vi "Read_Data_file_old.vi"(0 "Results file":path, 1 "Read Channel Names only":bool, 3 "Add Extra Channels?":bool, 5 "Template File":path, 8 "Read Results file only?":bool) -> (10 "Row numbers":i32[](array[numeric]), 11 "Template File Out":path, 12 "Filetype":string, 13 "EOF?":bool, 14 "Results file Out":path, 15 "String Before":string, 16 "Ch names Out":string[](array[string]), 17 "Channel Values Out":string[][](array[string]), 18 "String After":string, 19 "mark after read (chars.)":i32)   [LabVIEW 2010]
uses:
  Results_plotter_Global.vi
  Globals/Meas_global.vi
panel:
  out "Case":string
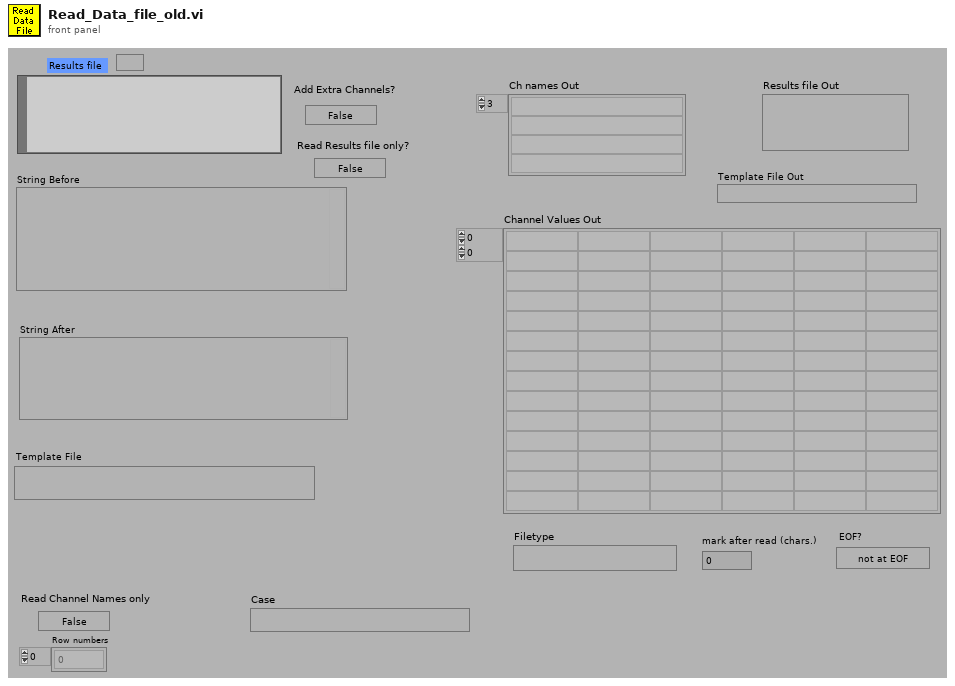
[diagram p1: front panel]
types:
  T1 = enum32{"existing file", "new file", "new or existing file", "existing dir", "new dir", "new or existing dir", "existing file (use LLBs)", "new file (use LLBs)", "new or existing file (use LLBs)", "new or existing file or directory (use LLBs)"}
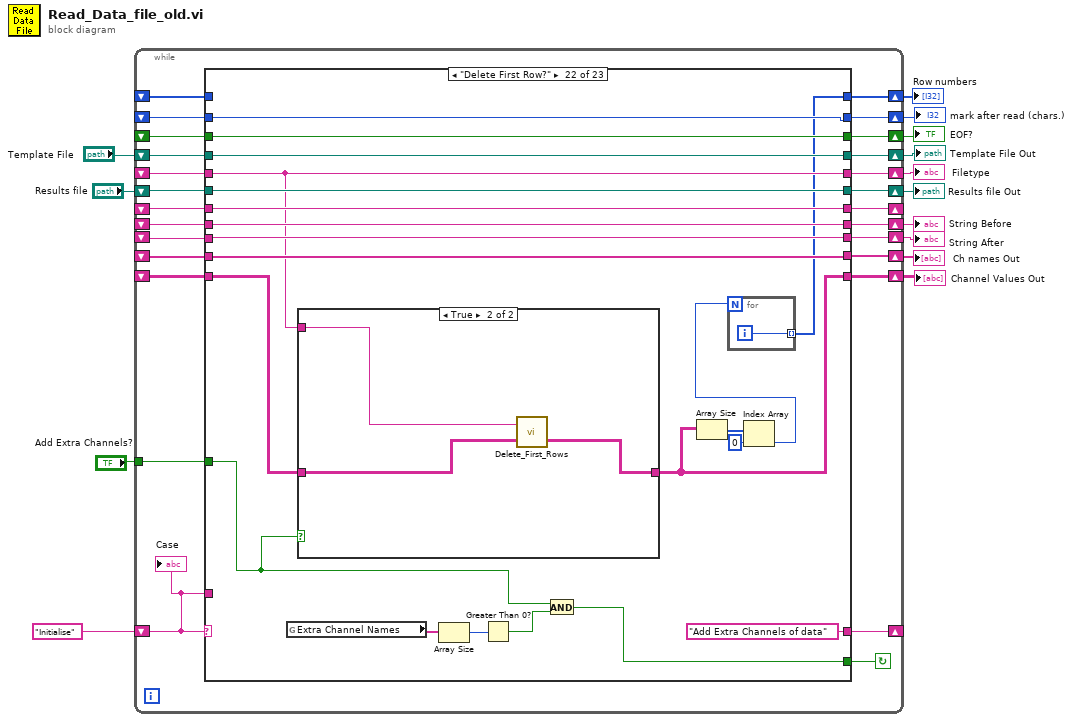
[diagram p0: block diagram]
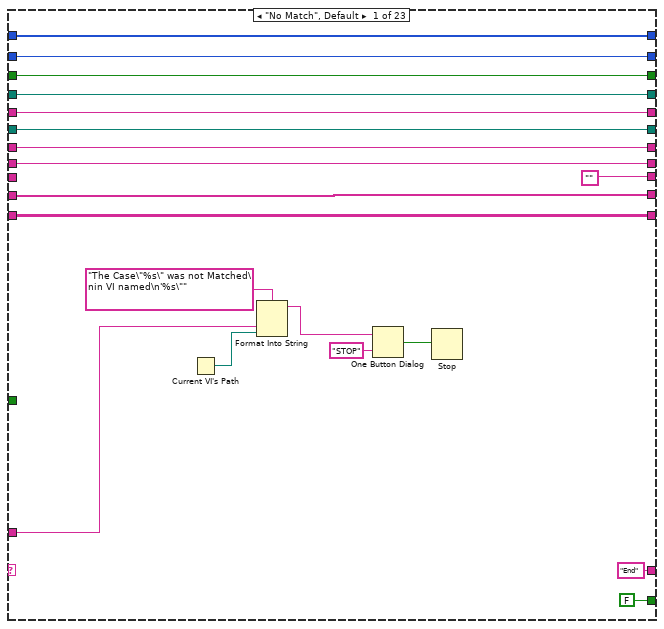
[diagram p2: hidden frame]
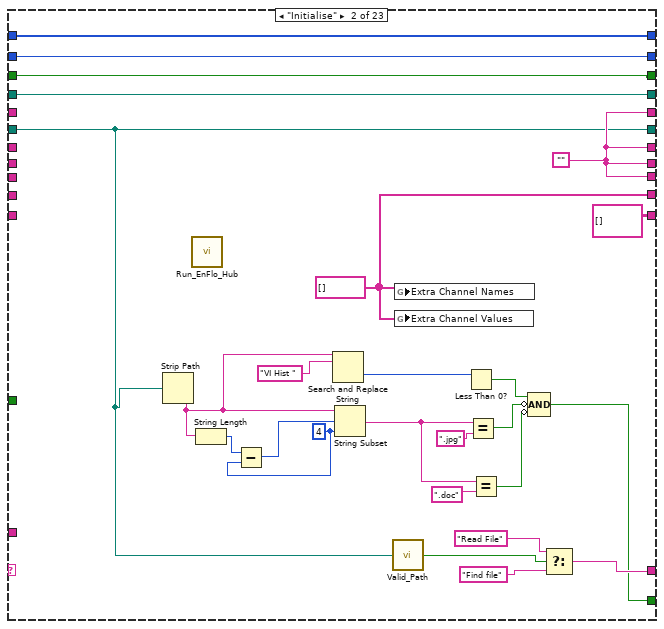
[diagram p3: hidden frame]
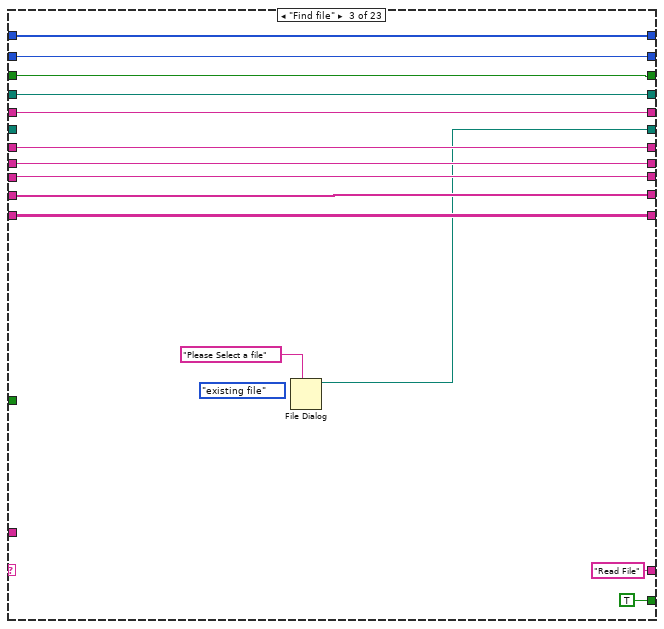
[diagram p4: hidden frame]
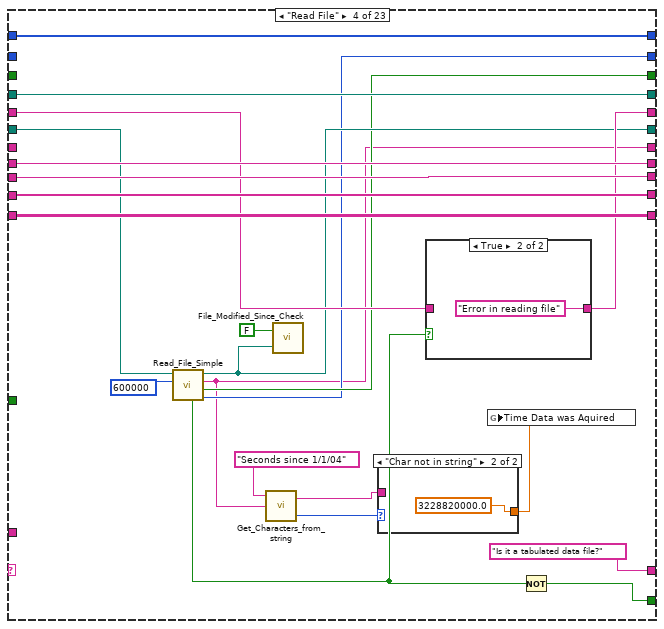
[diagram p5: hidden frame]
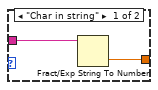
[diagram p6: hidden frame]
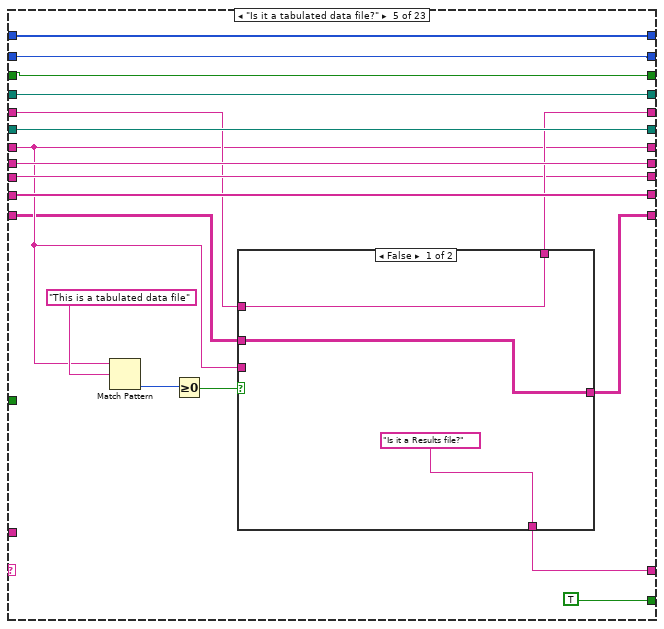
[diagram p8: hidden frame]
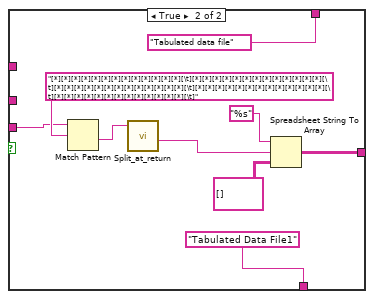
[diagram p9: hidden frame]
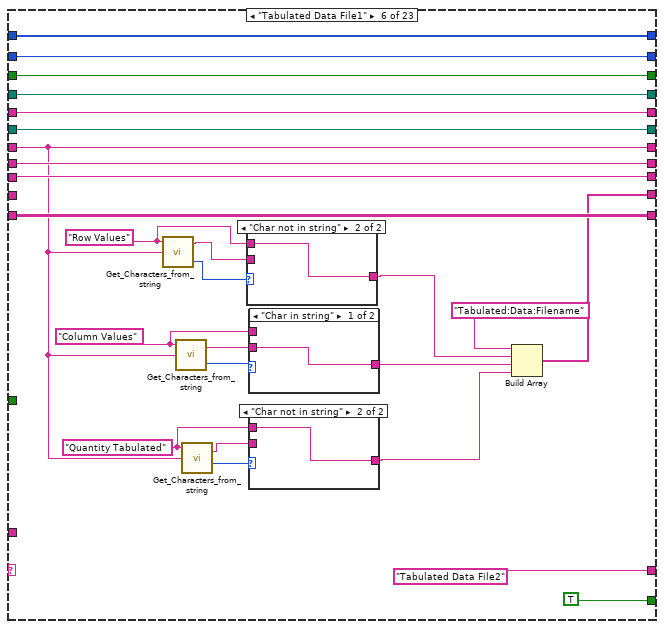
[diagram p10: hidden frame]
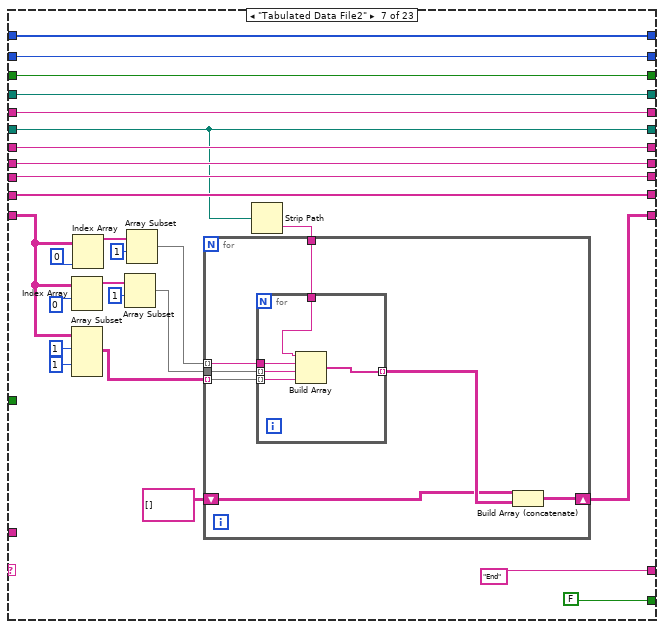
[diagram p14: hidden frame]
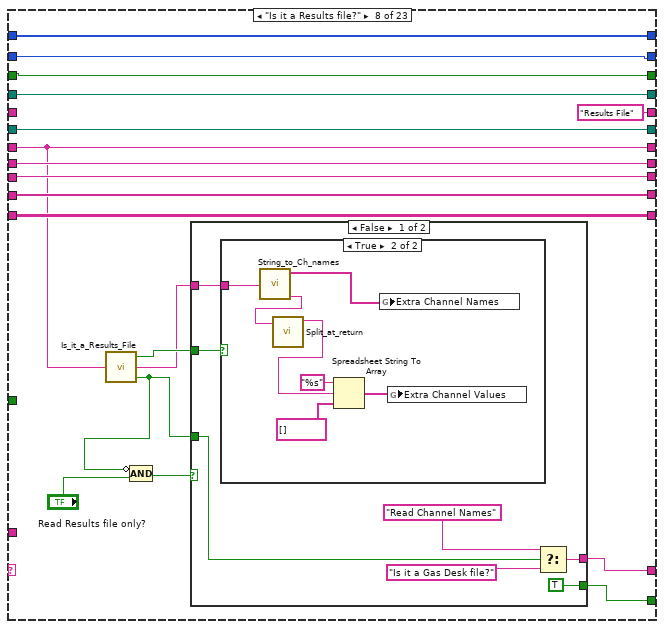
[diagram p15: hidden frame]
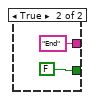
[diagram p17: hidden frame]
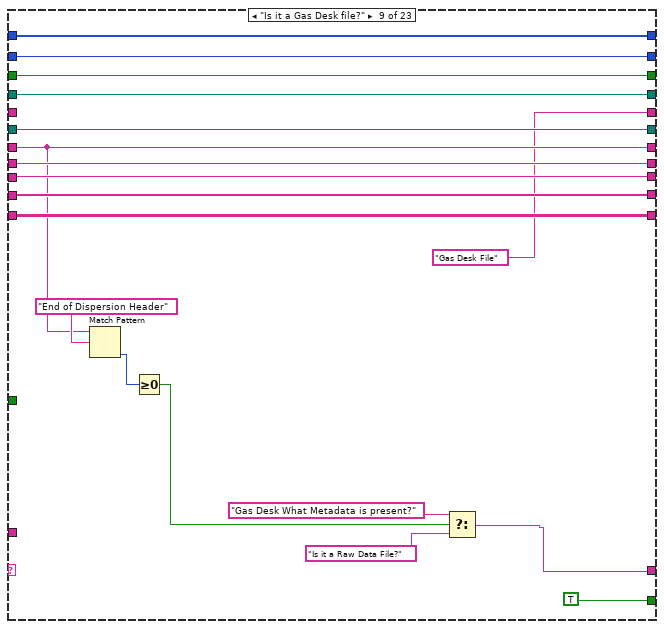
[diagram p18: hidden frame]
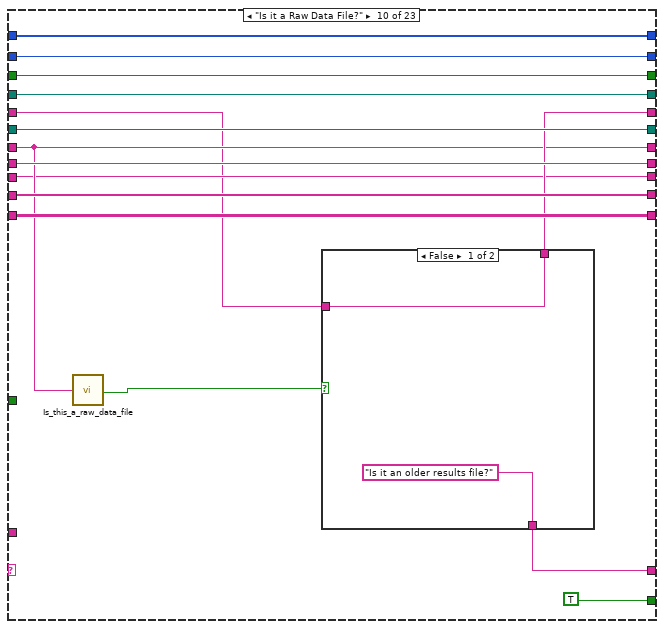
[diagram p19: hidden frame]
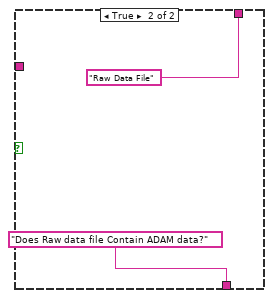
[diagram p20: hidden frame]
diagram:
  n1 = while {
    tunnel: "Add Extra Channels?" -> [w23]
    shift-left: _ -> [w27]
    shift-right: [w26] -> w13
    shift-left: "Results file" -> [w29]
    shift-right: [w28] -> w11
    shift-left: _ -> [w31]
    shift-right: [w30] -> w6
    shift-left: _ -> [w24]
    shift-right: [w32] -> w8
    shift-left: _ -> [w33]
    shift-right: [w34] -> _
    shift-left: "Initialise" -> [w37]
    shift-right: [w35] -> _
    shift-left: _ -> [w25]
    shift-right: [w39] -> w9
    shift-left: _ -> [w36]
    shift-right: [w40] -> w10
    shift-right: [w22] -> w5
    shift-left: "Template File" -> [w21]
    shift-right: [w19] -> w3
    shift-left: _ -> [w20]
    shift-right: [w18] -> w2
    shift-left: _ -> [w17]
    shift-right: [w15] -> w1
    shift-left: _ -> [w16]
    stop <- w38 continue-if-true
    n2 = case shown="\"Delete First Row?\"" w37 {
      tunnel: [w52 w83 w97 w119 w143 w163 w214 w244 w278 w293 w314 w339 w366 w387 w426 w454 w467 w529 w552 w588 w614 w646 w665] -> w40
      tunnel: [w51 string[][] [] ("Channel Values") w96 w118 w131 w181 w203 w243 w277 w292 w313 w338 w365 w386 w425 w453 w475 w535 w577 w587 w609 w635 w661] -> w39
      tunnel: [FALSE ("Results File?") w72 TRUE ("Results File?") w115 TRUE ("Results File?") TRUE ("Results File?") FALSE ("Results File?") w235 TRUE ("Results File?") TRUE ("Results File?") TRUE ("Results File?") w324 w358 TRUE ("Results File?") TRUE ("Results File?") TRUE ("Results File?") w461 TRUE ("Results File?") TRUE ("Results File?") FALSE ("Results File?") TRUE ("Results File?") w640 FALSE ("Results File?")] -> w38
      tunnel: w37 -> [w54 _ _ _ _ _ _ _ _ _ _ _ _ _ _ _ _ _ _ _ _ _ _]
      tunnel: w36 -> [w52 _ w97 w119 w143 _ w214 w244 w278 w293 w314 w339 w366 w387 w426 w454 _ w529 w553 w592 w614 w646 w668]
      tunnel: ["End" w84 "Read File" "Is it a tabulated data file?" w138 "Tabulated Data File2" ("f") "End" ("f") w242 w265 w287 w308 "Read Channel Names" ("f") "Read Channel Names" ("f") w372 "Read Channel Names" ("f") "Read Channel Names" ("f") w465 "Does template file exist?" ("f") w572 "End" ("f") "Delete First Row?" ("f") "Add Extra Channels of data" ("f") "End" ("f")] -> w35
      tunnel: [w49 w81 w94 w101 w132 w174 w210 w237 w271 w285 w303 w333 w354 w374 w404 w437 w468 w530 w576 w593 w607 w648 w670] -> w34
      tunnel: w33 -> [w49 _ w94 _ w132 w174 w210 w237 w271 w285 w303 w333 w361 w373 w404 w437 w470 w530 w576 w593 w607 w648 w670]
      tunnel: [w48 w81 w93 w117 w141 w179 w213 w238 w274 w290 w311 w336 w363 w383 w422 w451 w469 w527 w575 w596 w613 w651 w674] -> w32
      tunnel: w31 -> [_ _ w92 w116 w137 w177 w211 w240 w275 w284 w307 w335 _ w384 w423 w452 w474 w534 w574 w595 w612 w650 w673]
      tunnel: ["" w81 w92 w116 w137 w177 w211 w240 w275 w284 w307 w335 w351 w384 w423 w452 w474 w534 w574 w595 w612 w650 w673] -> w30
      tunnel: w29 -> [w47 w65 _ w112 w142 w180 w193 w241 w276 w291 w312 w337 w364 w385 w424 w431 w473 w533 w570 w591 w606 w647 w669]
      tunnel: [w47 w65 w91 w108 w142 w180 w193 w241 w276 w291 w312 w337 w364 w385 w424 w431 w473 w533 w570 w591 w606 w647 w669] -> w28
      tunnel: w27 -> [w45 _ w89 w113 w136 w176 w209 _ _ w283 w306 _ w357 w371 w420 w449 w472 w532 w573 w590 w603 w645 w672]
      tunnel: [w45 w81 w89 w114 w139 w176 w209 "Results File" "Gas Desk File" w288 w309 w323 w357 w371 w420 w449 w472 w532 w573 w590 w603 w645 w672] -> w26
      tunnel: w25 -> [w51 _ w96 w118 w130 w181 w202 w243 w277 w292 w313 w338 w365 w386 w425 w453 w475 w535 w577 _ _ w644 w663]
      tunnel: w24 -> [w48 _ w93 w117 w141 w179 w213 w238 w274 w290 w311 w336 w363 w383 w422 w451 _ w527 w575 w596 w613 w651 w674]
      tunnel: w23 -> [_ _ _ _ _ _ _ _ _ _ _ w325 _ _ _ _ _ _ _ _ _ w639 _]
      tunnel: [w44 w71 w88 w107 w129 w159 w191 w231 w264 w282 w301 w322 w348 w370 w402 w430 w463 w525 w555 w586 w602 w638 w660] -> w22
      tunnel: w21 -> [w44 w71 w88 w107 w129 w159 w191 w231 w264 w282 w301 w322 w348 w370 w402 w430 w463 w525 w555 w585 w602 w638 w660]
      tunnel: w20 -> [w42 w69 w86 _ w127 w157 w189 w229 w262 w280 w299 w320 w346 w368 w400 w428 w462 w524 w564 w584 w601 w636 w658]
      tunnel: [w42 w69 w86 w106 w127 w157 w189 w229 w262 w280 w299 w320 w346 w368 w400 w428 w462 w524 w564 w584 w600 w636 w658] -> w19
      tunnel: [w43 w70 w87 w105 w128 w158 w190 w230 w263 w281 w300 w321 w347 w369 w401 w429 w458 w523 w563 w583 w599 w637 w659] -> w18
      tunnel: w17 -> [w43 w70 w87 _ w128 w158 w190 w230 w263 w281 w300 w321 w347 w369 w401 w429 w459 w523 w563 w583 w599 w637 w659]
      tunnel: [w41 w68 w85 w104 w126 w156 w188 w228 w261 w279 w298 w319 w345 w367 w399 w427 w455 w522 w562 w582 w598 w631 w657] -> w15
      tunnel: w16 -> [w41 w68 w85 w104 w126 w156 w188 w228 w261 w279 w298 w319 w345 w367 w399 w427 w455 w522 w562 _ w598 _ w657]
      frame "No Match", Default {
        n3 = Current VI's Path() -> (path=w55:path)
        n4 = Format Into String(format string="The Case\"%s\" was not Matched\nin VI named\n'%s\"" ("Format String"), w54, w55) -> (resulting string=w58:string)  [unwired: 2 in, 1 out]
        n5 = One Button Dialog(message=w58, button name ("OK")="STOP") -> (true=w56:bool)
        n6 = Stop(stop? (T)=w56) -> ()
      }
      frame "Initialise" {
        w79 = 4 ("length (rest)")
        w81 = ""
        w83 = string[] [] ("Extra Channel Names")
        n7 = Strip Path(path=w65) -> (name=w77:string)  [unwired: 1 out]
        n8 = call "Run_EnFlo_Hub.vi"() -> ()  [unwired: 8 in]
        n9 = String Length(string=w77) -> (length=w80:i32)
        n10 = Subtract(x=w80, y=w79) -> (x-y=w78:i32)
        n11 = Search and Replace String(input string=w77, search string="VI Hist ") -> (offset past replacement=w75:i32)  [unwired: 6 in, 3 out]
        n12 = String Subset(string=w77, offset (0)=w78, length (rest)=w79) -> (substring=w62:string)
        n13 = call "Valid_Path.vi"("Filename"=w65) -> ("Valid Path?"=w64:bool)
        n14 = global write "Results_plotter_Global.vi" "Extra Channel Names"(w83) -> ()
        n15 = global write "Results_plotter_Global.vi" "Extra Channel Values"(w83) -> ()
        n16 = Less Than 0?(x=w75) -> (x < 0?=w73:bool)
        n17 = Equal?(x=w62, y=".jpg") -> (x = y?=w74:bool)
        n18 = Equal?(x=w62, y=".doc") -> (x = y?=w61:bool)
        n19 = Compound Arithmetic op=AND(w73, invert w74, invert w61) -> (w72:bool)
        n20 = Select(t="Read File", s=w64, f="Find file") -> (s? t:f=w84:string)
      }
      frame "Find file" {
        (unwired) T1."existing file" ("select mode (2)")
        n21 = File Dialog(7:"Please Select a file" ("prompt")) -> (3:w91:path)  [unwired: 6 in, 3 out]
      }
      frame "Read File" {
        n22 = call "Read_File_Simple.vi"("Filename"=w112, "number of characters (all:-1)"=600000 ("count")) -> ("Error?"=w110:bool, "Filename Out"=w108:path, "string"=w101:string, "EOF?"=w106:bool, "mark after read (chars.)"=w105:i32)  [unwired: 3 in, 1 out]
        n23 = call "Get_Characters_from_string.vi"("Input string"=w101, "Variable name"="Seconds since 1/1/04") -> ("Status"=w99:enum16{"Char in string", "Char not in string"}, "Value"=w102:string)  [unwired: 1 in]
        n24 = call "File_Modified_Since_Check.vi"("Pathname"=w108, "Just Modified?"=FALSE) -> ()  [unwired: 1 out]
        n25 = case shown="\"Char not in string\"" w99 {
          tunnel: w102 -> [w122 _]
          tunnel: [w121 3228820000.0 ("y")] -> w100
          frame "Char in string" {
            n26 = Fract/Exp String To Number(string=w122) -> (number=w121:dbl)  [unwired: 3 in, 1 out]
          }
          frame "Char not in string" {
          }
        }
        n27 = case shown="True" w110 {
          tunnel: [w124 "Error in reading file"] -> w114
          tunnel: w113 -> [w124 _]
          frame False {
          }
          frame True {
          }
        }
        n28 = global write "Meas_global.vi" "Time Data was Aquired"(w100) -> ()
        n29 = Not(x=w110) -> (.not. x?=w115:bool)
      }
      frame "Is it a tabulated data file?" {
        n30 = Match Pattern(string=w132, regular expression="This is a tabulated data file") -> (offset past match=w135:i32)  [unwired: 1 in, 3 out]
        n31 = Greater Or Equal To 0?(x=w135) -> (x >= 0?=w134:bool)
        n32 = case shown="False" w134 {
          tunnel: [w146 "Tabulated data file"] -> w139
          tunnel: ["Is it a Results file?" "Tabulated Data File1" ("f")] -> w138
          tunnel: w136 -> [w146 _]
          tunnel: w132 -> [_ w152]
          tunnel: [w145 w149] -> w131
          tunnel: w130 -> [w145 _]
          frame False {
          }
          frame True {
            n33 = Match Pattern(string=w152, regular expression="[*][*][*][*][*][*][*][*][*][*][*][*][*][\t][*][*][*][*][*][*][*][*][*][*][*][*][*][\t][*][*][*][*][*][*][*][*][*][*][*][*][*][\t][*][*][*][*][*][*][*][*][*][*][*][*][*][\t][*][*][*][*][*][*][*][*][*][*][*][*][*][\t]" ("String")) -> (after substring=w148:string)  [unwired: 1 in, 3 out]
            n34 = call "Split_at_return.vi"("String"=w148) -> ("after substring"=w147:string)  [unwired: 1 in, 3 out]
            n35 = Spreadsheet String To Array(format string="%s", spreadsheet string=w147, array type (2D Dbl)=string[][] [] ("Channel Values")) -> (array=w149:string[][])  [unwired: 1 in]
          }
        }
      }
      frame "Tabulated Data File1" {
        w162 = "Row Values" ("Variable name")
        w161 = "Column Values" ("Variable name")
        w168 = "Quantity Tabulated" ("Variable name")
        n36 = call "Get_Characters_from_string.vi"("Input string"=w174, "Variable name"=w162) -> ("Status"=w166:enum16{"Char in string", "Char not in string"}, "Value"=w167:string)  [unwired: 1 in]
        n37 = call "Get_Characters_from_string.vi"("Input string"=w174, "Variable name"=w161) -> ("Status"=w173:enum16{"Char in string", "Char not in string"}, "Value"=w172:string)  [unwired: 1 in]
        n38 = call "Get_Characters_from_string.vi"("Input string"=w174, "Variable name"=w168) -> ("Status"=w170:enum16{"Char in string", "Char not in string"}, "Value"=w169:string)  [unwired: 1 in]
        n39 = case shown="\"Char not in string\"" w166 {
          tunnel: w167 -> [w184 _]
          tunnel: [w184 w185] -> w165
          tunnel: w162 -> [_ w185]
          frame "Char in string" {
          }
          frame "Char not in string" {
          }
        }
        n40 = case shown="\"Char in string\"" w173 {
          tunnel: w172 -> [w186 _]
          tunnel: [w186 w187] -> w171
          tunnel: w161 -> [_ w187]
          frame "Char in string" {
          }
          frame "Char not in string" {
          }
        }
        n41 = case shown="\"Char not in string\"" w170 {
          tunnel: w169 -> [w182 _]
          tunnel: [w182 w183] -> w164
          tunnel: w168 -> [_ w183]
          frame "Char in string" {
          }
          frame "Char not in string" {
          }
        }
        n42 = Build Array("Tabulated:Data:Filename", w165, w171, w164) -> (w163:string[])
      }
      frame "Tabulated Data File2" {
        n43 = Index Array(array=w202, index (row)=0) -> (element=w201:string[])  [unwired: 1 in]
        n44 = Array Subset(array=w202, index (row)=1 ("index"), index (col)=1 ("index")) -> (w205:string[][])  [unwired: 2 in]
        n45 = Index Array(array=w202, index (col)=0 ("index (row)")) -> (element=w197:string[])  [unwired: 1 in]
        n46 = Array Subset(array=w201, index=1) -> (w198:string[])  [unwired: 1 in]
        n47 = Array Subset(array=w197, index=1) -> (w196:string[])  [unwired: 1 in]
        n48 = Strip Path(path=w193) -> (name=w192:string)  [unwired: 1 out]
        n49 = for {
          tunnel: w196 -> [w221] mode=indexing
          tunnel: w198 -> [w220]
          tunnel: w205 -> [w219] mode=indexing
          shift-right: [w216] -> w203
          shift-left: string[][] [] -> [w217]
          tunnel: w192 -> [w215]
          n50 = for {
            tunnel: w221 -> [w226]
            tunnel: w220 -> [w225] mode=indexing
            tunnel: w219 -> [w224] mode=indexing
            tunnel: [w223] -> w218 mode=indexing
            tunnel: w215 -> [w222]
            n51 = Build Array(w222, w226, w225, w224) -> (w223:string[])
          }
          n52 = Build Array (concatenate)(w217, w218) -> (w216:string[][])
        }
      }
      frame "Is it a Results file?" {
        n53 = call "Is_it_a_Results_File.vi"("character string"=w237) -> ("Contain DB Header Info"=w236:bool, "Header String"=w227:string, "Results File?"=w233:bool)
        n54 = Compound Arithmetic op=AND(invert w233, "Read Results file only?") -> (w232:bool)
        n55 = case shown="False" w232 {
          tunnel: [w250 "End"] -> w242
          tunnel: w233 -> [w248 _]
          tunnel: w227 -> [w247 _]
          tunnel: w236 -> [w246 _]
          tunnel: [TRUE ("Results File?") FALSE ("Results File?")] -> w235
          frame False {
            n56 = case shown="True" w246 {
              tunnel: w247 -> [_ w254]
              frame False {
              }
              frame True {
                n57 = call "String_to_Ch_names.vi"("Spreadsheet string"=w254) -> ("Ch names"=w253:string[], "String After names"=w257:string)  [unwired: 2 out]
                n58 = call "Split_at_return.vi"("String"=w257) -> ("before substring"=w258:string)  [unwired: 1 in, 3 out]
                n59 = Spreadsheet String To Array(format string="%s", spreadsheet string=w258, array type (2D Dbl)=string[] [] ("Channel Values")) -> (array=w252:string[])  [unwired: 1 in]
                n60 = global write "Results_plotter_Global.vi" "Extra Channel Names"(w253) -> ()
                n61 = global write "Results_plotter_Global.vi" "Extra Channel Values"(w252) -> ()
              }
            }
            n62 = Select(t="Read Channel Names", s=w248, f="Is it a Gas Desk file?") -> (s? t:f=w250:string)
          }
          frame True {
          }
        }
      }
      frame "Is it a Gas Desk file?" {
        n63 = Match Pattern(string=w271, regular expression="End of Dispersion Header") -> (offset past match=w273:i32)  [unwired: 1 in, 3 out]
        n64 = Greater Or Equal To 0?(x=w273) -> (x >= 0?=w268:bool)
        n65 = Select(t="Gas Desk What Metadata is present?" ("f"), s=w268, f="Is it a Raw Data File?") -> (s? t:f=w265:string)
      }
      frame "Is it a Raw Data File?" {
        n66 = call "Is_this_a_raw_data_file.vi"("character string"=w285) -> ("Raw Dat File?"=w286:bool)  [unwired: 2 in]
        n67 = case shown="False" w286 {
          tunnel: [w294 "Raw Data File"] -> w288
          tunnel: ["Is it an older results file?" ("f") "Does Raw data file Contain ADAM data?" ("f")] -> w287
          tunnel: w283 -> [w294 _]
          frame False {
          }
          frame True {
          }
        }
      }
      frame "Is it an older results file?" {
        n68 = Match Pattern(string=w303, regular expression="Date of meas\tTime of meas") -> (offset past match=w304:i32)  [unwired: 1 in, 3 out]
        n69 = Greater Or Equal To 0?(x=w304) -> (x >= 0?=w302:bool)
        n70 = case shown="False" w302 {
          tunnel: [w316 "Older Results File"] -> w309
          tunnel: ["Is it a calibration file?" ("f") "Read Channel Names" ("f")] -> w308
          tunnel: w306 -> [w316 _]
          frame False {
          }
          frame True {
          }
        }
      }
      frame "Is it a calibration file?" {
        w332 = FALSE  # Show Dialog?
        n71 = call "2D_array_from_string.vi"("Show Dialog?"=w332, "Input string"=w333, "Array title"="Calib points label") -> ("2D data array"=w331:dbl[][])
        n72 = Array Size(array=w331) -> (size(s)=w330:i32[])
        n73 = Index Array(array=w330, index=0 ("Index")) -> (element=w328:i32)
        n74 = Greater Than 0?(x=w328) -> (x > 0?=w326:bool)
        n75 = case shown="True" w326 {
          tunnel: w325 -> [_ w344]
          tunnel: [TRUE ("Results File?") w343] -> w324
          tunnel: ["File with no header" "Calibration File"] -> w323
          frame False {
          }
          frame True {
            n76 = Not(x=w344) -> (.not. x?=w343:bool)
          }
        }
      }
      frame "Does Raw data file Contain ADAM data?" {
        w349 = "\r"
        w352 = "Raw data header Start"
        n77 = Match Pattern(string=w361, regular expression=w352) -> (before substring=w355:string, after substring=w350:string)  [unwired: 1 in, 2 out]
        n78 = Match Pattern(string=w355, regular expression="[*][*][*][*][*][*][*][*][*][*][*][*][*][*][*][*][*][*][*][*][*]" ("String")) -> (before substring=w354:string)  [unwired: 1 in, 3 out]
        n79 = Concatenate Strings(w349, "************************", w349, w352, w350) -> (w351:string)
        n80 = String Length(string=w355) -> (length=w360:i32)
        n81 = Greater?(x=w360, y=30) -> (0:w358:bool)
      }
      frame "Gas Desk What Metadata is present?" {
        n82 = String Subset(string=w373, offset (0)=0, length (rest)=6 ("length")) -> (substring=w380:string)
        n83 = Equal?(x="******", y=w380) -> (x = y?=w378:bool)
        n84 = case shown="False" w378 {
          tunnel: [w389 "Gas Desk Read ADAM ch's Header"] -> w372
          tunnel: w373 -> [w388 _]
          frame False {
            w393 = "Data Base\tData Base\tData Base\t"
            n85 = String Length(string=w393) -> (length=w396:i32)
            n86 = String Subset(string=w388, offset (0)=0, length (rest)=w396) -> (substring=w394:string)
            n87 = Equal?(x=w393, y=w394) -> (x = y?=w392:bool)
            n88 = Select(t="Gas Desk DB Header Present", s=w392, f="Read Channel Names") -> (s? t:f=w389:string)
          }
          frame True {
          }
        }
        n89 = call "Fast_string_Replace.vi"("Replace match with:"="Suspect Pulse Width" ("regular expression"), "Input String"=w373, "regular expression"="Suspect \u0003Pulse Width ") -> ("Output String"=w374:string)  [unwired: 1 in, 1 out]
      }
      frame "Gas Desk DB Header Present" {
        w407 = string[] [] ("Channel Values")
        n90 = call "String_to_Ch_names.vi"("Spreadsheet string"=w404) -> ("Ch names"=w419:string[], "String After names"=w408:string)  [unwired: 2 out]
        n91 = call "Split_at_return.vi"("String"=w408) -> ("before substring"=w410:string, "after substring"=w411:string)  [unwired: 1 in, 2 out]
        n92 = call "Split_at_return.vi"("String"=w411) -> ("after substring"=w412:string)  [unwired: 1 in, 3 out]
        n93 = call "String_to_Ch_names.vi"("Spreadsheet string"=w412) -> ("Ch names"=w418:string[], "String After names"=w413:string)  [unwired: 2 out]
        n94 = call "Split_at_return.vi"("String"=w413) -> ("after substring"=w415:string)  [unwired: 1 in, 3 out]
        n95 = call "Split_at_return.vi"("String"=w415) -> ("before substring"=w416:string)  [unwired: 1 in, 3 out]
        n96 = Spreadsheet String To Array(format string="%s", spreadsheet string=w410, array type (2D Dbl)=w407) -> (array=w406:string[])  [unwired: 1 in]
        n97 = Spreadsheet String To Array(format string="%s", spreadsheet string=w416, array type (2D Dbl)=w407) -> (array=w417:string[])  [unwired: 1 in]
        n98 = Build Array (concatenate)(w418, w419) -> (w398:string[])
        n99 = Build Array (concatenate)(w417, w406) -> (w405:string[])
        n100 = global write "Results_plotter_Global.vi" "Extra Channel Values"(w405) -> ()
        n101 = global write "Results_plotter_Global.vi" "Extra Channel Names"(w398) -> ()
      }
      frame "Gas Desk Read ADAM ch's Header" {
        n102 = call "Split_at_return.vi"("String"=w437) -> ("after substring"=w445:string)  [unwired: 1 in, 3 out]
        n103 = call "String_to_Ch_names.vi"("Spreadsheet string"=w445) -> ("Ch names"=w433:string[], "String After names"=w446:string)  [unwired: 2 out]
        n104 = call "Split_at_return.vi"("String"=w446) -> ("after substring"=w447:string)  [unwired: 1 in, 3 out]
        n105 = call "Split_at_return.vi"("String"=w447) -> ("before substring"=w444:string)  [unwired: 1 in, 3 out]
        n106 = Spreadsheet String To Array(format string="%s", spreadsheet string=w444, array type (2D Dbl)=string[] [] ("Channel Values")) -> (array=w438:string[])  [unwired: 1 in]
        n107 = Strip Path(path=w431) -> (stripped path=w440:path, name=w439:string)
        n108 = Path To String(path=w440) -> (string=w441:string)
        n109 = Build Array (concatenate)("Original:Results:Filename", "Original:Results:Filepath", w433) -> (w432:string[])
        n110 = Build Array (concatenate)(w439, w441, w438) -> (w436:string[])
        n111 = global write "Results_plotter_Global.vi" "Extra Channel Names"(w432) -> ()
        n112 = global write "Results_plotter_Global.vi" "Extra Channel Values"(w436) -> ()
      }
      frame "Read Channel Names" {
        n113 = case shown="\"Older Results File\"" w472 {
          tunnel: [w483 w497 w506 0 0] -> w456
          tunnel: [w482 w496 w510 w515 w520] -> w466
          tunnel: w470 -> [w481 w498 w509 w518 w520]
          tunnel: [w480 w504 "Is Raw Data Filename Present?" ("f") w513 w519] -> w465
          tunnel: "Does template file exist?" ("f") -> [w480 w504 _ w513 w519]
          frame "Results File" {
            n114 = Match Pattern(string=w481, regular expression="[*][*][*][*][*][*][*][*][*][*][*][*][*][\t][*][*][*][*][*][*][*][*][*][*][*][*][*][\t][*][*][*][*][*][*][*][*][*][*][*][*][*][\t][*][*][*][*][*][*][*][*][*][*][*][*][*][\t][*][*][*][*][*][*][*][*][*][*][*][*][*][\t]" ("String")) -> (after substring=w486:string, offset past match=w484:i32)  [unwired: 1 in, 2 out]
            n115 = call "Split_at_return.vi"("String"=w486) -> ("after substring"=w482:string, "offset past match"=w485:i32)  [unwired: 1 in, 2 out]
            n116 = Add(x=w484, y=w485) -> (x+y=w483:i32)
          }
          frame "Older Results File" {
            w491 = "\r"
            n117 = Match Pattern(string=w498, regular expression="Date of meas\tTime of meas") -> (before substring=w502:string, match substring=w495:string, offset past match=w499:i32)  [unwired: 1 in, 1 out]
            n118 = Reverse String(1:w502) -> (0:w501:string)
            n119 = String Length(string=w495) -> (length=w494:i32)
            n120 = Match Pattern(string=w501, regular expression=w491) -> (after substring=w500:string, offset past match=w492:i32)  [unwired: 1 in, 2 out]
            n121 = Match Pattern(string=w500, regular expression=w491) -> (after substring=w490:string, offset past match=w493:i32)  [unwired: 1 in, 2 out]
            n122 = Match Pattern(string=w490, regular expression=w491) -> (offset past match=w489:i32)  [unwired: 1 in, 3 out]
            n123 = Compound Arithmetic op=ADD(invert w494, w499, invert w493, invert w492, invert w489, 1 ("value")) -> (w497:i32)
            n124 = Search/Split String(string=w498, offset (0)=w497) -> (match + rest of string=w496:string)  [unwired: 1 in, 2 out]
          }
          frame "Gas Desk File" {
            n125 = Match Pattern(string=w509, regular expression="End of Dispersion Header") -> (after substring=w512:string, offset past match=w507:i32)  [unwired: 1 in, 2 out]
            n126 = call "Split_at_return.vi"("String"=w512) -> ("after substring"=w510:string, "offset past match"=w508:i32)  [unwired: 1 in, 2 out]
            n127 = Add(x=w508, y=w507) -> (x+y=w506:i32)
          }
          frame "Raw Data File" {
            n128 = Search/Split String(string=w518, offset (0)=37 ("y")) -> (match + rest of string=w517:string)  [unwired: 1 in, 2 out]
            n129 = call "Split_at_return.vi"("String"=w517) -> ("after substring"=w515:string)  [unwired: 1 in, 3 out]
          }
          frame "File with no header", Default {
          }
        }
        n130 = call "String_to_Ch_names.vi"("Spreadsheet string"=w466) -> ("Ch names"=w467:string[], "Title length (Bytes)"=w457:i32, "String After names"=w468:string)  [unwired: 1 out]
        n131 = case shown="True" "Read Channel Names only" {
          tunnel: w459 -> [w476 _]
          tunnel: [w476 w477] -> w458
          tunnel: w457 -> [_ w479]
          tunnel: w456 -> [_ w478]
          frame False {
          }
          frame True {
            n132 = Add(x=w478, y=w479) -> (x+y=w477:i32)
          }
        }
        n133 = String Subset(string=w470, offset (0)=0, length (rest)=w456) -> (substring=w469:string)
        n134 = Not(x="Read Channel Names only") -> (.not. x?=w461:bool)
      }
      frame "Is Raw Data Filename Present?" {
        w526 = "Raw:Data:Filename"
        n135 = Search 1D Array(1D array=w529, element=w526) -> (index of element=w528:i32)  [unwired: 1 in]
        n136 = case shown="-1" w528 {
          tunnel: w527 -> [_ w549]
          tunnel: w526 -> [_ w543]
          frame 0, Default {
          }
          frame -1 {
            n137 = global read "Results_plotter_Global.vi" "Extra Channel Names"() -> (w544:string[])
            n138 = global read "Results_plotter_Global.vi" "Extra Channel Values"() -> (w542:string[])
            n139 = Concatenate Strings("Raw data Directory", "\t") -> (w546:string)
            n140 = Match Pattern(string=w549, regular expression=w546) -> (after substring=w545:string)  [unwired: 1 in, 3 out]
            n141 = call "Split_at_return.vi"("String"=w545) -> ("before substring"=w538:string)  [unwired: 1 in, 3 out]
            n142 = Build Array (concatenate)(w544, w543) -> (w540:string[])
            n143 = global write "Results_plotter_Global.vi" "Extra Channel Names"(w540) -> ()
            n144 = Match Pattern(string=w538, regular expression="\t") -> (before substring=w537:string)  [unwired: 1 in, 3 out]
            n145 = Build Array (concatenate)(w542, w537) -> (w541:string[])
            n146 = global write "Results_plotter_Global.vi" "Extra Channel Values"(w541) -> ()
          }
        }
      }
      frame "Does template file exist?" {
        n147 = global read "Results_plotter_Global.vi" "Extra Channel Names"() -> (w571:string[])
        n148 = while {
          shift-right: [w580] -> w559
          shift-left: _ -> [w581]
          stop <- TRUE stop-if-true
          n149 = Increment(x=w581) -> (x+1=w580:dbl)
        }
        n150 = call "Common_Extra_Chs.vi"() -> ("Common Extra Channels"=w561:string[])
        n151 = call "Valid_Path.vi"("Filename"=w555) -> ("Valid Path?"=w554:bool)
        n152 = Path to Array of Strings(0:w570) -> (2:w569:string[])  [unwired: 1 out]
        n153 = global read "Results_plotter_Global.vi" "Extra Channel Values"() -> (w567:string[])
        n154 = Build Array (concatenate)(w571, w561) -> (w551:string[])
        n155 = Reverse 1D Array(array=w569) -> (reversed array=w568:string[])
        n156 = call "Update_Ch_Names.vi"("Ch Name in"=w551) -> ("Ch Name Out"=w550:string[])
        n157 = Array Subset(array=w568, length=5) -> (w566:string[])  [unwired: 1 in]
        n158 = Number To Decimal String(number=w559) -> (decimal integer string=w558:string)  [unwired: 1 in]
        n159 = Select(t="Read Values using Template", s=w554, f="Entire string to 2D array") -> (s? t:f=w572:string)
        n160 = Build Array (concatenate)(w567, w566, w558) -> (w565:string[])
        n161 = global write "Results_plotter_Global.vi" "Extra Channel Names"(w550) -> ()
        n162 = call "Update_Ch_Names.vi"("Ch Name in"=w553) -> ("Ch Name Out"=w552:string[])
        n163 = global write "Results_plotter_Global.vi" "Extra Channel Values"(w565) -> ()
      }
      frame "Read Values using Template" {
        n164 = call "Filter_on_template_file_new.vi"("Filetype"=w590, "Filename"=w591, "End Of File already Reached?"=w584, "Start of data (bytes)"=w583, "Data string"=w593, "Channel Names In"=w592, "Template File"=w585) -> ("Data Out"=w589:string[][], "Channel Names Out"=w588:string[], "Row numbers"=w582:i32[], "Template File-write"=w586:path)  [unwired: 1 in]
        n165 = call "Surface_modularity.vi"("Data in"=w589, "Channel names"=w588) -> ("Data out"=w587:string[][])  [unwired: 1 in]
      }
      frame "Entire string to 2D array" {
        n166 = case shown="\"False\", Default" w603 {
          tunnel: [w620 w630] -> w608
          tunnel: w607 -> [w619 w630]
          tunnel: w606 -> [w618 _]
          tunnel: w601 -> [w616 w629]
          tunnel: [w617 w629] -> w600
          tunnel: w599 -> [w615 _]
          frame "False", Default {
            n167 = case shown="False" w616 {
              tunnel: [w624 w628] -> w620
              tunnel: w619 -> [w626 w628]
              tunnel: w618 -> [w623 _]
              tunnel: [w622 w627] -> w617
              tunnel: w616 -> [_ w627]
              tunnel: w615 -> [w621 _]
              frame False {
                n168 = call "Read_Characters_From_File.ph.vi"("file path (dialog if empty)"=w623, "start of read offset (chars.: 0)"=w621) -> ("character string"=w625:string, "EOF?"=w622:bool)  [unwired: 4 in, 2 out]
                n169 = Concatenate Strings(w626, w625) -> (w624:string)
              }
              frame True {
              }
            }
          }
          frame "Raw Data File" {
          }
        }
        n170 = Spreadsheet String To Array(format string="%s", spreadsheet string=w608, array type (2D Dbl)=string[][] [] ("Channel Values")) -> (array=w609:string[][])  [unwired: 1 in]
      }
      frame "Delete First Row?" {
        n171 = global read "Results_plotter_Global.vi" "Extra Channel Names"() -> (w643:string[])
        n172 = case shown="True" w639 {
          tunnel: w645 -> [_ w656]
          tunnel: w644 -> [w653 w655]
          tunnel: [w653 w654] -> w635
          frame False {
          }
          frame True {
            n173 = call "Delete_First_Rows.vi"("Data In"=w655, "File Type"=w656) -> ("Data Out"=w654:string[][])  [unwired: 1 out]
          }
        }
        n174 = Array Size(array=w643) -> (size(s)=w642:i32)
        n175 = Greater Than 0?(x=w642) -> (x > 0?=w641:bool)
        n176 = And(x=w639, y=w641) -> (x .and. y?=w640:bool)
        n177 = Array Size(array=w635) -> (size(s)=w634:i32[])
        n178 = Index Array(array=w634, index=0) -> (element=w632:i32)
        n179 = for {
          N: w632 -> [_]
          tunnel: [w652] -> w631 mode=indexing
          i -> [w652]
        }
      }
      frame "Add Extra Channels of data" {
        n180 = global read "Results_plotter_Global.vi" "Extra Channel Names"() -> (w666:string[])
        n181 = global read "Results_plotter_Global.vi" "Extra Channel Values"() -> (w664:string[])
        n182 = for {
          tunnel: w666 -> [w683] mode=indexing
          shift-right: [w681] -> w662
          shift-left: string[] [] -> [w682]
          shift-right: [w684] -> w665
          shift-left: w668 -> [w679]
          tunnel: w664 -> [w680] mode=indexing
          n183 = Search 1D Array(1D array=w679, element=w683) -> (index of element=w685:i32)  [unwired: 1 in]
          n184 = case shown="-1" w685 {
            tunnel: w679 -> [w687 w693]
            tunnel: [w687 w692] -> w684
            tunnel: w683 -> [_ w691]
            tunnel: w682 -> [w686 w690]
            tunnel: [w686 w689] -> w681
            tunnel: w680 -> [_ w688]
            frame 0, Default {
            }
            frame -1 {
              n185 = Build Array (concatenate)(w693, w691) -> (w692:string[])
              n186 = Build Array (concatenate)(w690, w688) -> (w689:string[])
            }
          }
        }
        n187 = for {
          tunnel: w663 -> [w676] mode=indexing
          tunnel: w662 -> [w678]
          tunnel: [w677] -> w661 mode=indexing
          n188 = Build Array (concatenate)(w676, w678) -> (w677:string[])
        }
      }
    }
    "Case" <- w37
  }
  "Filetype" <- w13
  "Results file Out" <- w11
  "Ch names Out" <- w10
  "Channel Values Out" <- w9
  "String Before" <- w8
  "String After" <- w6
  "Template File Out" <- w5
  "EOF?" <- w3
  "mark after read (chars.)" <- w2
  "Row numbers" <- w1
